vi "Configure IR.vi"(0 "VISA resource name":refnum<visa-resource-name>, 1 "Test Voltage (V)":string, 2 "Pre-Check Delay (s)":string, 3 "Dwell Time (s)":string, 4 "Min IR Limit (ohm)":string, 5 "Max IR Limit (ohm)":string, 6 "DUT Type I":string(combo)="Isolated DUT", 7 "error in (no error)":errorcluster, 9 "DUT Type II":string(combo)="Resistive DUT", 11 "Command Terminator":bool=TRUE) -> (20 "VISA resource name out":refnum<visa-resource-name>, 21 "Command Output":string, 25 "Error Message":string, 26 "Error Code":i32, 27 "error out":errorcluster)   [LabVIEW 2010, in "VITREK V7X.lvlib"]
doc: "Configures the <b>IR</b> input.\n\n<b>Note:</b> please refer to the instrument manual for the <b>IR</b> input specification.\n- When field 7 is GND - Grounded DUT, no matter what's in field 8, error code 3 will be reported by ERR?"
uses:
  VITREK V7X.lvlib
panel:
  # "Yes\n\nNo"
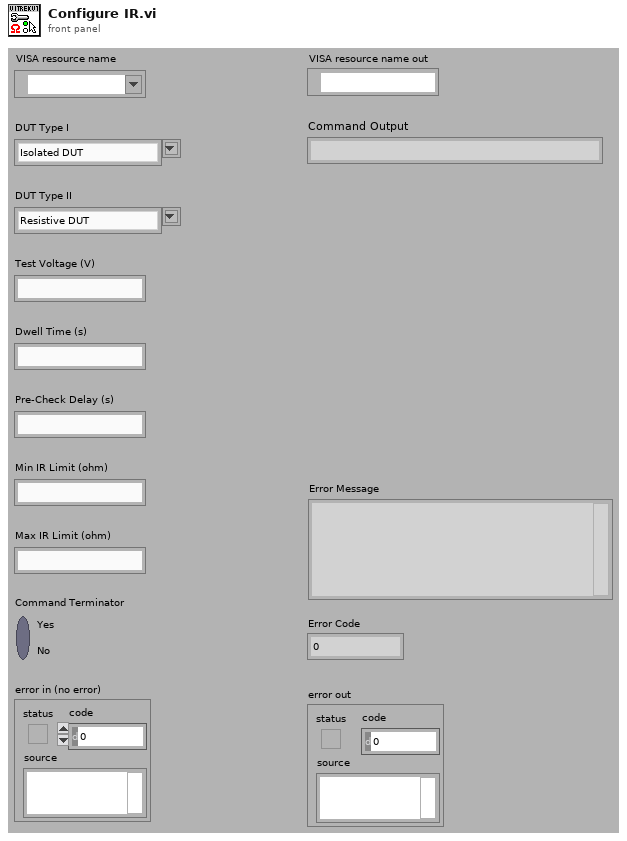
[diagram p1: front panel]
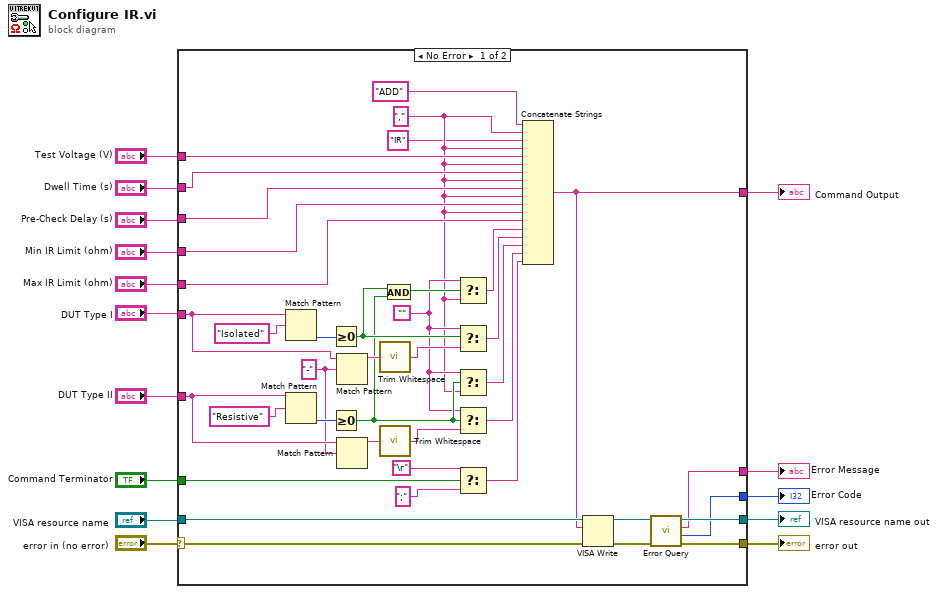
[diagram p0: block diagram]
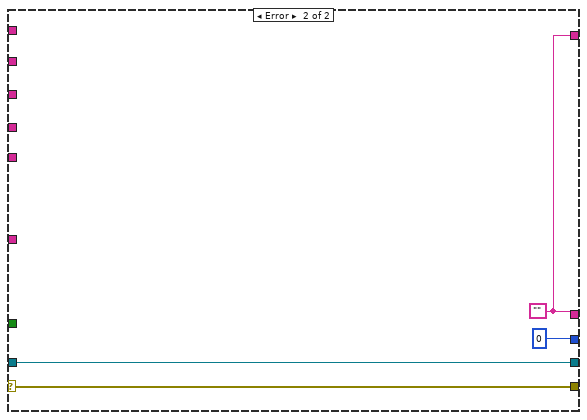
[diagram p2: hidden frame]
diagram:
  n1 = case shown="No Error" "error in (no error)" {
    selector: "error in (no error)" -> [w50 w58]
    tunnel: "VISA resource name" -> [w55 w59]
    tunnel: [w43 w56] -> w14
    tunnel: [w52 w59] -> w13
    tunnel: [w51 w58] -> w12
    tunnel: "Test Voltage (V)" -> [w49 _]
    tunnel: "Dwell Time (s)" -> [w48 _]
    tunnel: "Pre-Check Delay (s)" -> [w47 _]
    tunnel: "Min IR Limit (ohm)" -> [w46 _]
    tunnel: "Max IR Limit (ohm)" -> [w45 _]
    tunnel: "Command Terminator" -> [w40 _]
    tunnel: "DUT Type I" -> [w35 _]
    tunnel: "DUT Type II" -> [w28 _]
    tunnel: [w17 0] -> w2
    tunnel: [w16 w56] -> w1
    frame No Error {
      w19 = "-"
      w22 = ""
      w21 = ","
      n2 = Match Pattern(string=w35, regular expression="Isolated") -> (offset past match=w36:i32)  [unwired: 1 in, 3 out]
      n3 = Match Pattern(string=w28, regular expression="Resistive") -> (offset past match=w31:i32)  [unwired: 1 in, 3 out]
      n4 = Greater Or Equal To 0?(x=w36) -> (x >= 0?=w27:bool)
      n5 = Greater Or Equal To 0?(x=w31) -> (x >= 0?=w23:bool)
      n6 = Match Pattern(string=w35, regular expression=w19) -> (before substring=w34:string)  [unwired: 1 in, 3 out]
      n7 = Match Pattern(string=w28, regular expression=w19) -> (before substring=w30:string)  [unwired: 1 in, 3 out]
      n8 = call <vilib>:"Trim Whitespace.vi"("string"=w34) -> ("trimmed string"=w33:string)  [unwired: 1 in]
      n9 = call <vilib>:"Trim Whitespace.vi"("string"=w30) -> ("trimmed string"=w29:string)  [unwired: 1 in]
      n10 = And(x=w27, y=w23) -> (x .and. y?=w26:bool)
      n11 = Select(t=w22, s=w26, f=w21) -> (s? t:f=w41:string)
      n12 = Select(t=w22, s=w27, f=w33) -> (s? t:f=w42:string)
      n13 = Select(t=w22, s=w23, f=w21) -> (s? t:f=w20:string)
      n14 = Select(t=w22, s=w23, f=w29) -> (s? t:f=w24:string)
      n15 = Select(t="\r", s=w40, f=";") -> (s? t:f=w25:string)
      n16 = Concatenate Strings("ADD", w21, "IR", w21, w49, w21, w48, w21, w47, w21, w46, w21, w45, w41, w42, w20, w24, w25) -> (w43:string)
      n17 = VISA Write(VISA resource name=w55, write buffer=w43, error in (no error)=w50) -> (VISA resource name out=w54:refnum<visa-resource-name>, error out=w53:errorcluster)  [unwired: 1 out]
      n18 = call "Error Query.vi"("error in (no error)"=w53, "VISA resource name"=w54) -> ("error out"=w51:errorcluster, "Error Code"=w17:i32, "Error Message"=w16:string, "VISA resource name out"=w52:refnum<visa-resource-name>)  [unwired: 6 in]
    }
    frame Error {
      w56 = ""
    }
  }
  "VISA resource name out" <- w13
  "error out" <- w12
  "Command Output" <- w14
  "Error Code" <- w2
  "Error Message" <- w1
